vi "Dialog_Clear Calibration.vi"() -> (3 "Clear Type Requested (Galvo; Reso; Both; None)":string)   [LabVIEW 2012]
panel:
  in  "Cancel Button":bool
  in  "OK Button":bool
  in  "Select the calibration files to clear":T1
  # "This action will clear all your previous calibrations!"
  # "Click 'Cancel' to abort"
  # "Click 'Confirm' to proceed"
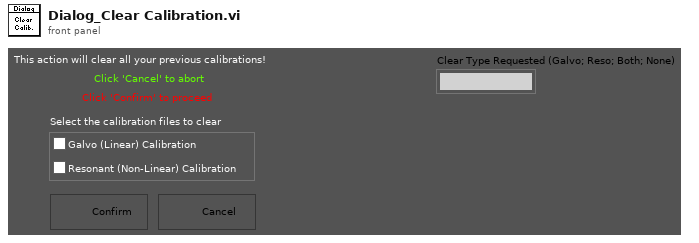
[diagram p1: front panel]
types:
  T1 = cluster{"Resonant (Non-Linear) Calibration":bool, "Galvo (Linear) Calibration":bool}
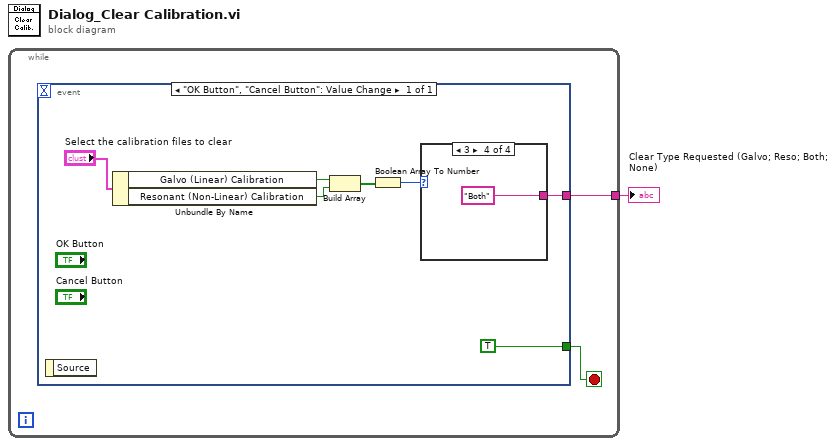
[diagram p0: block diagram]
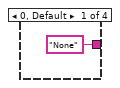
[diagram p2: hidden frame]
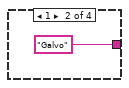
[diagram p3: hidden frame]
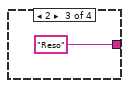
[diagram p4: hidden frame]
diagram:
  n1 = while {
    tunnel: [w2] -> w1
    stop <- w3 stop-if-true
    n2 = event shown="[0] \"OK Button\", \"Cancel Button\": Value Change" {
      selector: _ -> [_]
      dyn-events: _ -> [_]
      timeout: _ -> [_]
      tunnel: [TRUE] -> w3
      tunnel: [w4] -> w2
      event "OK Button", "Cancel Button": Value Change {
        n3 = event-data() -> ()  [unwired: 1 in, 1 out]
        n4 = Unbundle By Name("Select the calibration files to clear") -> ("Galvo (Linear) Calibration"=w6:bool, "Resonant (Non-Linear) Calibration"=w5:bool)
        n5 = Build Array(w6, w5) -> (w8:bool[])
        n6 = Boolean Array To Number(Boolean array=w8) -> (number=w7:u32)
        n7 = case shown="3" w7 {
          tunnel: ["None" "Galvo" "Reso" "Both"] -> w4
          frame 0, Default {
          }
          frame 1 {
          }
          frame 2 {
          }
          frame 3 {
          }
        }
      }
    }
  }
  "Clear Type Requested (Galvo; Reso; Both; None)" <- w1
